vi "Engine-DestroyWindow.vi"(8 "error in (no error)":errorcluster, 11 "Window in":refnum<class "Window.lvclass">) -> (0 "error out":errorcluster, 3 "Window out":refnum<class "Window.lvclass">)   [LabVIEW 2020, in "GLF.lvlib" / "Window.lvclass"]
uses:
  Window.lvclass
  Window.lvclass/Window.ctl
  <vilib>/Saukko/LV SDL3/Sources/SDL3/Video/Video.lvlib
  <vilib>/Saukko/LV SDL3/Sources/SDL3/Video/WindowID--integer.ctl
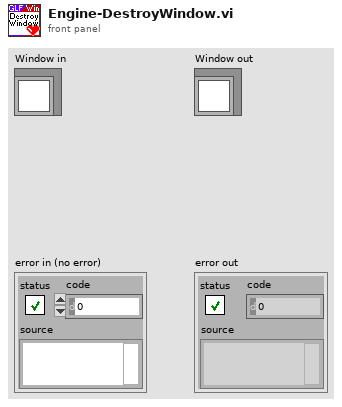
[diagram p1: front panel]
types:
  T1 = typedef "SDL3.lvlib/Video.lvlib/WindowID--integer.ctl" = u32
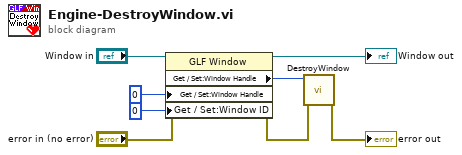
[diagram p0: block diagram]
diagram:
  n1 = property class="GLF Window"(reference="Window in", error in="error in (no error)", "Get / Set:Window Handle"=i64 0 ("SDL_Window *"), "Get / Set:Window ID"=T1 0 ("Window ID")) -> (reference out=→"Window out":refnum<class "Window.lvclass">, error out=w2:errorcluster, "Get / Set:Window Handle"=w7:i64)
  n2 = call <vilib>:"DestroyWindow.vi"("No Error"=w2, "Window [SDL_Window*]"=w7) -> ("Error Out"=→"error out":errorcluster)  [unwired: 9 in]
